vi "tx poulse host.vi"() -> ()   [LabVIEW 2021]
uses:
  <instrlib>/niUsrpRio/Config/v1/Host/Private/LO Source.ctl
  <vilib>/FPGAPlugInAG/USRP 294xR; 295xR 200 MSps/niLvFpga_Open_USRP 294xR; 295xR 200 MSps.vi
  <vilib>/rvi/interface/common/dynamic/niFpgaDynamicAddResources.vi
  <vilib>/Utility/error.llb/Error Cluster From Error Code.vi
  <vilib>/rvi/errors/niLvFpgaAdjustHostInterfaceError.vi
  <vilib>/rvi/interface/common/niFpgaWaitOnOcc.vi
  <vilib>/FPGAPlugInAG/Dynamic/niLvFpga_Close_Dynamic.vi
  <vilib>/rvi/interface/nirviOpenFPGA/nirviOpenFPGA.xnode
  FPGA Bitfiles/niUsrpRio200_XcvrTime.lvbitx
  <vilib>/rvi/interface/nirviMethod/nirviMethod.xnode
  <vilib>/rvi/interface/nirviReadWriteControl/nirviReadWriteControl.xnode
  <vilib>/rvi/interface/nirviCloseFPGA/nirviCloseFPGA.xnode
  <instrlib>/niUsrpRio/Config/v1/Host/niUsrpRio Config v1 Host.lvlib
  NiFpgaLv.dll
  <vilib>/rvi/interface/Simulation/niFpgaSimulationCallBeginRW.vi
  <vilib>/FPGAPlugInAG/Dynamic/niLvFpga_WriteFifo_Dynamic.vi
  <vilib>/rvi/errors/niLvFpgaMergeErrorWithErrorCode.vi
  <vilib>/FPGAPlugInAG/Dynamic/niLvFpga_ConfigureFifo_Dynamic.vi
panel:
  out "tx free":bool[](array[boolean])
  in  "analog file 3":path=path "C:/Users/NI/Documents/chaim/chaim_rx/chaim_data/good morning.wav"
  in  "analog file 2":path=path "C:/Users/NI/Documents/chaim/chaim_rx/chaim_data/good morning.wav"
  in  "analog file 1":path=path "C:/Users/NI/Documents/chaim/chaim_rx/chaim_data/good morning.wav"
  out "# pulse sent to FPGA":dbl
  out "pulse Tx by FPGA":u32
  out "fpga clock":dbl
  in  "tdms pulse istraction file path":path=path "C:/Users/NI/Documents/chaim/chaim_rx/chaim_data/pulses.tdms"
  in  "stop":bool
  in  "gain 0":dbl=-20.0 format="%#_6p"
  in  "Tx. frequency 0":dbl=2000000000.0 format="%#_6p"
  # "pulse transmitter"
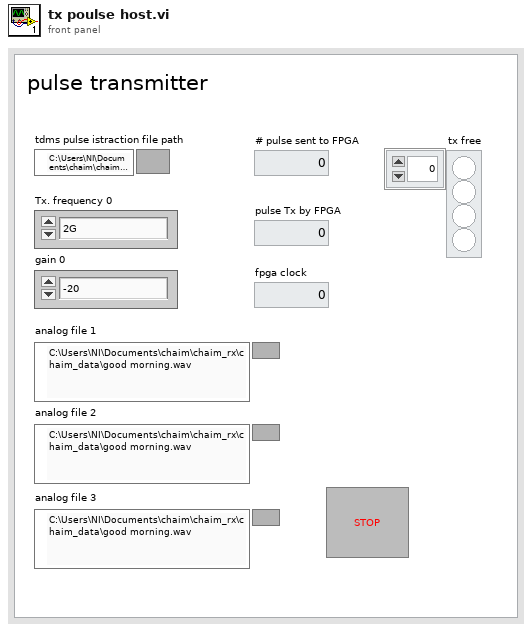
[diagram p1: front panel]
types:
  T1 = enum16{"open", "open or create", "create or replace", "create", "open (read-only)"}
  T2 = typedef "niUsrpRio Config v1 Host.lvlib/LO Source.ctl" = enum16{"Internal", "Companion", "External", "Reimport"}
  T3 = typedef "niUsrpRio Config v1 Host.lvlib/niUsrpRio Session.ctl" = cluster{"FPGA Interface":refnum<k20>, "RIO Interface Number":u32, "Data Clock Rate":u32, "FPGA Data Clock Rate":u32, "Global Settings Register Bus":T4, "Radio 0 Settings Register Bus":T4, "Radio 1 Settings Register Bus":T4, "Radio Settings Bus Semaphore":T5, "DB Queues":T6[], "Characterization Data Valid?":bool, "EEPROM Header":T7, "Device Data Header":T8, "EEPROM Characterization Header":T9, "Characterization Data":T10[], "FPGA Current Version":u32, "FPGA Oldest Compatible Version":u32, "Fixed Logic Current Version":u32, "Fixed Logic Oldest Compatible Version":u32, "FPGA Radio Settings Bus Current Version":u32, "FPGA Radio Settings Bus Oldest Compatible Version":u32, "FPGA Board Config Current Version":u32, "FPGA Board Config Oldest Compatible Version":u32, "Daughterboard Clock Rate":u32, "daughterboard configuration session handles":u64[]}
  T4 = typedef "niInstr Register Bus v0 Host.lvlib/Register Bus Session.ctl" = refnum<queue>
  T5 = typedef "Semaphore RefNum" = refnum<k1>
  T6 = typedef "niUsrpRio Config v1 Host.lvlib/DB Queue Reference.ctl" = refnum<queue>
  T7 = typedef "niUsrpRio Config v1 Host.lvlib/EEPROM Header.ctl" = cluster{"Checksum":u32, "Product Code":u16, "Hardware Current Version":u16, "Hardware Oldest Compatible Version":u16, "EEPROM Map Current Version":u16, "EEPROM Map Oldest Compatible Version":u16, "User Password":string, "Pointer to Factory Header":u32, "Pointer to User Header":u32, "Recommended Interval":u16, "Number of Reserved Bytes":i32, "Number of Daughterboards":u8, "Daughterboard IDs":u16[], "Daughterboard Serial Numbers":string[]}
  T8 = typedef "niUsrpRio Config v1 Host.lvlib/EEPROM Device Data Header.ctl" = cluster{"Checksum":u32, "Number of Channels":u8, "Number of Gain Settings":u16[], "Pointer to Characterization Data":u32[], "Number of Reserved Bytes":i32, "Number of Frequencies":u16[]}
  T9 = typedef "niUsrpRio Config v1 Host.lvlib/EEPROM Characterization Header.ctl" = cluster{"Checksum":u32, "Date":timestamp, "Temperature":sgl, "Misc. Info":string, "Pointer to Device Data Header":u32, "Number of Reserved Bytes":i32}
  T10 = typedef "niUsrpRio Config v1 Host.lvlib/Characterization Data.ctl" = cluster{"Gains[dB]":dbl[], "Frequencies [Hz]":dbl[], "IQ Imbalance Table":T11[], "Measured Gains[dB]":dbl[][]}
  T11 = typedef "niUsrpRio Config v1 Host.lvlib/IQ Imbalance.ctl" = cluster{"Gain Imbalance [linear]":dbl, "Phase Imbalance [radians]":dbl, "Offset":cdb}
  T12 = cluster{"gain I":fxp<+/-,24,3>, "gain Q":fxp<+/-,24,3>}
  T13 = typedef "niInstr DSP v1 Shared.lvlib/IQ Impairments.ctl" = cluster{"inline gain I":fxp<+/-,18,1>, "inline gain Q":fxp<+/-,18,1>, "cross gain I":fxp<+/-,18,1>, "cross gain Q":fxp<+/-,18,1>, "pre-gain offset I":fxp<+/-,18,1>, "pre-gain offset Q":fxp<+/-,18,1>, "post-gain offset I":fxp<+/-,18,1>, "post-gain offset Q":fxp<+/-,18,1>}
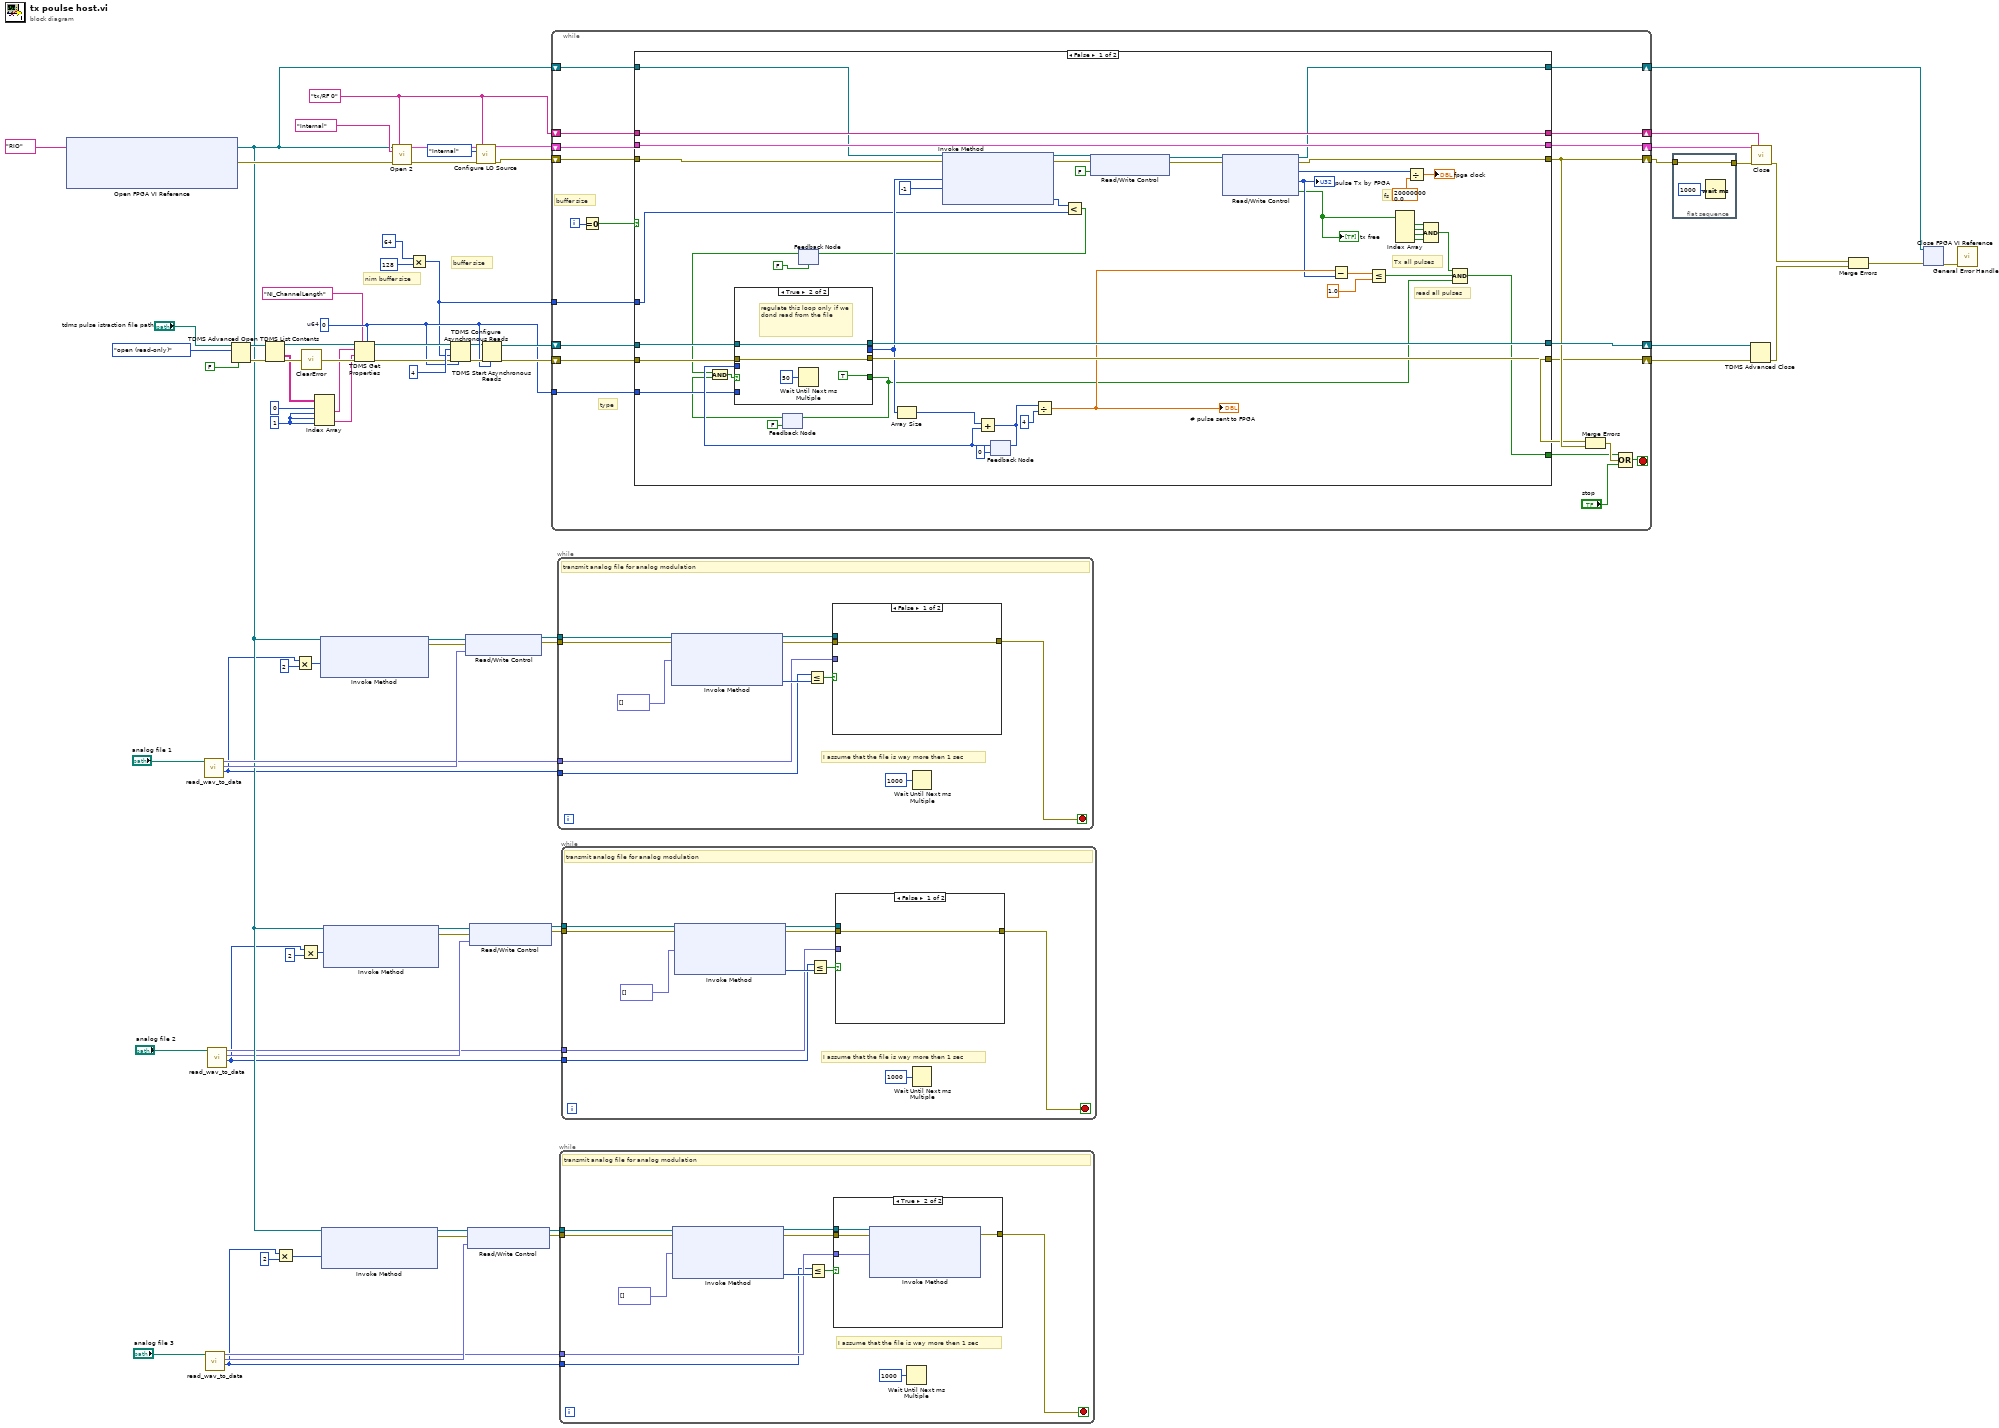
[diagram p0: block diagram]
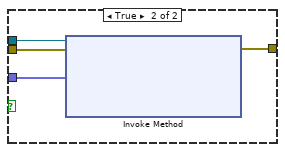
[diagram p3: hidden frame]
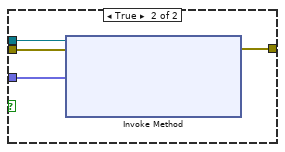
[diagram p4: hidden frame]
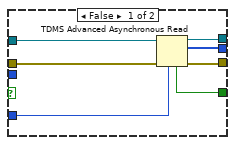
[diagram p5: hidden frame]
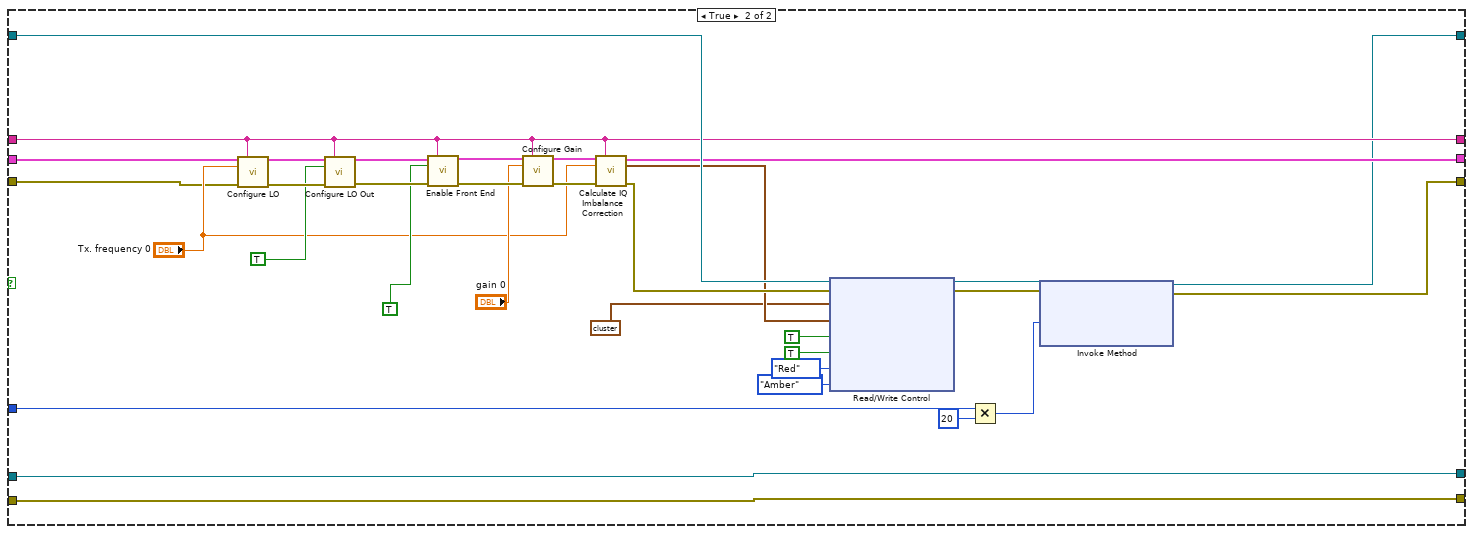
[diagram p6: hidden frame]
diagram:
  w46 = 1 ("disabled index (col)")
  w42 = u64 0  # u64
  w73 = "tx/RF 0" ("scope")
  # "buffer size"
  # "nim buffer size"
  n1 = xnode ("Open FPGA VI Reference")("resource name"=tag "RIO") -> ("FPGA VI Reference Out"=w15:refnum<k20>, "error out"=w39:errorcluster)  [unwired: 1 in]
  n2 = call "read_wav_to_data.vi"("path"="analog file 1") -> ("sampels on file"=w3:i32, "UP SAMPLE RATE"=w29:fxp<+,48,1>, "wav file out"=w28:fxp<+/-,18,1>[])  [unwired: 8 in]
  n3 = call "read_wav_to_data.vi"("path"="analog file 3") -> ("sampels on file"=w5:i32, "UP SAMPLE RATE"=w8:fxp<+,48,1>, "wav file out"=w7:fxp<+/-,18,1>[])  [unwired: 8 in]
  n4 = call "read_wav_to_data.vi"("path"="analog file 2") -> ("sampels on file"=w6:i32, "UP SAMPLE RATE"=w14:fxp<+,48,1>, "wav file out"=w11:fxp<+/-,18,1>[])  [unwired: 8 in]
  n5 = TDMS Advanced Open(6:FALSE ("Disable Buffering? (T)"), 10:T1."open (read-only)" ("Operation"), 11:"tdms pulse istraction file path") -> (0:w56:errorcluster, 3:w49:refnum<k34>)  [unwired: 2 in, 1 out]
  n6 = TDMS List Contents(4:w56, 7:w49) -> (0:w54:errorcluster, 1:w45:string[][], 3:w50:refnum<k34>)  [unwired: 1 in, 1 out]
  n7 = Multiply(x=w5, y=2) -> (x*y=w18:i32)
  n8 = Multiply(x=w3, y=2) -> (x*y=w32:i32)
  n9 = Multiply(x=w6, y=2) -> (x*y=w23:i32)
  n10 = call <vilib>:"ClearError.vi"("error in (no error)"=w54) -> ("error out"=w57:errorcluster)
  n11 = Index Array(array=w45, index (row) #1=0 ("index (row)"), index (col) #1=w46, index (row) #2=w46, index (col) #2=w46) -> (element #1=w44:string, element #2=w43:string)
  n12 = xnode ("Invoke Method")("FPGA VI Reference In"=w15, "Requested Depth"=w32) -> ("FPGA VI Reference Out"=w31:refnum<k20>, "error out"=w30:errorcluster)  [unwired: 1 in, 1 out]
  n13 = xnode ("Invoke Method")("FPGA VI Reference In"=w15, "Requested Depth"=w18) -> ("FPGA VI Reference Out"=w10:refnum<k20>, "error out"=w9:errorcluster)  [unwired: 1 in, 1 out]
  n14 = xnode ("Invoke Method")("FPGA VI Reference In"=w15, "Requested Depth"=w23) -> ("FPGA VI Reference Out"=w13:refnum<k20>, "error out"=w12:errorcluster)  [unwired: 1 in, 1 out]
  n15 = TDMS Get Properties(5:w42, 7:"NI_ChannelLength" ("property name"), 8:w57, 9:w43, 10:w44, 11:w50) -> (0:w55:errorcluster, 3:w48:refnum<k34>)  [unwired: 4 out]
  n16 = call <instrlib>:"Open 2.vi"("fpga ref"=w15, "scope"=w73, "Reference Frequency Source"="Internal", "error in"=w39) -> ("niUsrpRio Session (out)"=w65:T3, "error out"=w75:errorcluster)  [unwired: 10 in]
  n17 = Multiply(x=u32 64, y=u32 128 ("buffer size")) -> (x*y=w35:u32)
  n18 = TDMS Configure Asynchronous Reads(6:w42, 8:w55, 9:w35, 10:u32 4 ("Number of Buffers (4)"), 11:w48) -> (0:w59:errorcluster, 3:w41:refnum<k34>)  [unwired: 1 in]
  n19 = xnode ("Read/Write Control")("FPGA VI Reference In"=w31, "error in"=w30, "UP SAMPLE RATE"=w29) -> ("FPGA VI Reference Out"=w27:refnum<k20>, "error out"=w26:errorcluster)
  n20 = xnode ("Read/Write Control")("FPGA VI Reference In"=w10, "error in"=w9, "UP SAMPLE RATE 3"=w8) -> ("FPGA VI Reference Out"=w17:refnum<k20>, "error out"=w16:errorcluster)
  n21 = xnode ("Read/Write Control")("FPGA VI Reference In"=w13, "error in"=w12, "UP SAMPLE RATE 2"=w14) -> ("FPGA VI Reference Out"=w24:refnum<k20>, "error out"=w25:errorcluster)
  n22 = call <instrlib>:"Configure LO Source.vi"("niUsrpRio Session"=w65, "scope"=w73, "lo source"=LO_Source."Internal", "error in"=w75) -> ("niUsrpRio Session (out)"=w72:T3, "error out"=w71:errorcluster)  [unwired: 10 in]
  n23 = TDMS Start Asynchronous Reads(6:w42, 8:w59, 11:w41) -> (0:w51:errorcluster, 3:w52:refnum<k34>)  [unwired: 1 in]
  n24 = while {
    shift-right: [w82] -> w2
    shift-left: w71 -> [w95]
    shift-right: [w93] -> w70
    shift-left: w72 -> [w96]
    shift-right: [w92] -> w66
    shift-left: w15 -> [w94]
    shift-right: [w90] -> w69
    shift-left: w73 -> [w91]
    shift-right: [w85] -> w64
    shift-left: w52 -> [w87]
    shift-right: [w81] -> w63
    shift-left: w51 -> [w86]
    tunnel: w42 -> [w84]
    tunnel: w35 -> [w83]
    i -> [w88]
    stop <- w78 stop-if-true
    # "buffer size"
    # "type"
    n25 = Equal To 0?(x=w88) -> (x = 0?=w89:bool)
    n26 = case shown="False" w89 {
      tunnel: w96 -> [w142 w175]
      tunnel: w95 -> [w136 w174]
      tunnel: w94 -> [w135 w173]
      tunnel: [w142 w171] -> w93
      tunnel: [w111 w161] -> w92
      tunnel: [w110 w160] -> w82
      tunnel: w91 -> [w143 w170]
      tunnel: [w143 w170] -> w90
      tunnel: w87 -> [w134 w165]
      tunnel: w86 -> [w133 w164]
      tunnel: [w132 w165] -> w85
      tunnel: [w131 w164] -> w81
      tunnel: w84 -> [w125 _]
      tunnel: w83 -> [w122 w159]
      tunnel: [w104 _] -> w77
      frame False {
        # "fs"
        # "read all pulses"
        # "Tx all pulses"
        n27 = feedback #1(FALSE ("end of file?")) -> (w121:bool)
        n28 = feedback #2(FALSE) -> (w120:bool)
        n29 = Compound Arithmetic op=AND(w120, w121) -> (w117:bool)
        n30 = feedback #3(u32 0) -> (w129:u32)
        n31 = case shown="True" w117 {
          tunnel: w134 -> [w150 w154]
          tunnel: w133 -> [w145 w153]
          tunnel: [w149 w154] -> w132
          tunnel: [w146 w153] -> w131
          tunnel: [w147 _] -> w130
          tunnel: [w148 TRUE ("end of file?")] -> w103
          tunnel: w129 -> [_ _]
          tunnel: w125 -> [w144 _]
          frame False {
            n32 = TDMS Advanced Asynchronous Read(6:w144, 8:w145, 11:w150) -> (0:w146:errorcluster, 2:w147:u64[], 3:w149:refnum<k34>, 4:w148:bool)
          }
          frame True {
            # "regulate this loop only if we dond read from the file"
            n33 = Wait Until Next ms Multiple(millisecond multiple=u32 50) -> ()  [unwired: 1 out]
          }
        }
        n34 = feedback-in #1(w103) -> ()
        n35 = Array Size(array=w130) -> (size(s)=w127:i32)
        n36 = xnode ("Invoke Method")("FPGA VI Reference In"=w135, "error in"=w136, "Data"=w130, "Timeout (ms)"=-1) -> ("FPGA VI Reference Out"=w139:refnum<k20>, "error out"=w140:errorcluster, "Empty Elements Remaining"=w123:u32)
        n37 = Add(x=w127, y=w129) -> (x+y=w116:u32)
        n38 = feedback-in #3(w116) -> ()
        n39 = Divide(x=w116, y=u32 4) -> (x/y=w109:dbl)
        "# pulse sent to FPGA" <- w109
        n40 = Less?(x=w123, y=w122) -> (x < y?=w119:bool)
        n41 = feedback-in #2(w119) -> ()
        n42 = xnode ("Read/Write Control")("FPGA VI Reference In"=w139, "error in"=w140, "reset system clock"=FALSE) -> ("FPGA VI Reference Out"=w138:refnum<k20>, "error out"=w137:errorcluster)
        n43 = xnode ("Read/Write Control")("FPGA VI Reference In"=w138, "error in"=w137) -> ("FPGA VI Reference Out"=w111:refnum<k20>, "error out"=w110:errorcluster, "fpga clock"=w113:u64, "pulse transmitted"=w108:u32, "tx free"=w102:bool[])
        "pulse Tx by FPGA" <- w108
        "tx free" <- w102
        n44 = Subtract(x=w109, y=w108) -> (x-y=w107:dbl)
        n45 = Less Or Equal?(x=w107, y=1.0) -> (x <= y?=w105:bool)
        n46 = Index Array(array=w102) -> (element #1=w101:bool, element #2=w100:bool, element #3=w99:bool, element #4=w98:bool)  [unwired: 4 in]
        n47 = Divide(x=w113, y=200000000.0) -> (x/y=→"fpga clock":dbl)
        n48 = Compound Arithmetic op=AND(w101, w100, w99, w98) -> (w97:bool)
        n49 = Compound Arithmetic op=AND(w97, w105, w103) -> (w104:bool)
      }
      frame True {
        n50 = call <instrlib>:"Configure LO.vi"("niUsrpRio Session"=w175, "scope"=w170, "frequency"="Tx. frequency 0", "error in"=w174) -> ("niUsrpRio Session (out)"=w187:T3, "error out"=w186:errorcluster)  [unwired: 8 in, 2 out]
        n51 = call <instrlib>:"Configure LO Out.vi"("niUsrpRio Session"=w187, "scope"=w170, "enable"=TRUE ("enable 0"), "error in"=w186) -> ("niUsrpRio Session (out)"=w184:T3, "error out"=w181:errorcluster)  [unwired: 10 in]
        n52 = call <instrlib>:"Enable Front End.vi"("niUsrpRio Session"=w184, "scope"=w170, "enable"=TRUE ("enable 0 2"), "error in"=w181) -> ("niUsrpRio Session (out)"=w183:T3, "error out"=w182:errorcluster)  [unwired: 10 in]
        n53 = call <instrlib>:"Configure Gain.vi"("niUsrpRio Session"=w183, "scope"=w170, "gain"="gain 0", "error in"=w182) -> ("niUsrpRio Session (out)"=w178:T3, "error out"=w177:errorcluster)  [unwired: 9 in, 1 out]
        n54 = call <instrlib>:"Calculate IQ Imbalance Correction.vi"("niUsrpRio Session"=w178, "scope"=w170, "frequency"="Tx. frequency 0", "error in"=w177) -> ("niUsrpRio Session (out)"=w171:T3, "IQ imbalance correction"=w167:T13, "error out"=w172:errorcluster)  [unwired: 8 in, 1 out]
        n55 = xnode ("Read/Write Control")("FPGA VI Reference In"=w173, "error in"=w172, "tx.gain.0"=T12 {"gain I"=1.0, "gain Q"=1.0}, "tx.impairments.0"=w167, "reset system clock"=TRUE, "RF 0/Tx/Enable"=TRUE, "LED/RF 0/TX1 RX1"=enum8{"Off", "Green", "Red", "Amber"}."Red", "LED/RF 1/TX1 RX1"=enum8{"Off", "Green", "Red", "Amber"}."Amber") -> ("FPGA VI Reference Out"=w163:refnum<k20>, "error out"=w162:errorcluster)
        n56 = Multiply(x=w159, y=u32 20) -> (x*y=w157:u32)
        n57 = xnode ("Invoke Method")("FPGA VI Reference In"=w163, "error in"=w162, "Requested Depth"=w157) -> ("FPGA VI Reference Out"=w161:refnum<k20>, "error out"=w160:errorcluster)  [unwired: 1 out]
      }
    }
    n58 = Merge Errors(w81, w82) -> (w79:errorcluster)
    n59 = Compound Arithmetic op=OR(w77, w79, "stop") -> (w78:bool)
  }
  n60 = while {
    tunnel: w3 -> [w193]
    tunnel: w28 -> [w192]
    tunnel: w27 -> [w191]
    tunnel: w26 -> [w190]
    stop <- w189 stop-if-true
    # "I assume that the file is way more then 1 sec"
    # "transmit analog file for analog modulation"
    n61 = xnode ("Invoke Method")("FPGA VI Reference In"=w191, "error in"=w190, "Data"=fxp<+/-,18,1>[] []) -> ("FPGA VI Reference Out"=w198:refnum<k20>, "error out"=w197:errorcluster, "Empty Elements Remaining"=w195:u32)  [unwired: 1 in]
    n62 = Less Or Equal?(x=w193, y=w195) -> (x <= y?=w194:bool)
    n63 = case shown="False" w194 {
      tunnel: [w199 w203] -> w189
      tunnel: w198 -> [_ w202]
      tunnel: w197 -> [w199 w201]
      tunnel: w192 -> [_ w200]
      frame False {
      }
      frame True {
        n64 = xnode ("Invoke Method")("FPGA VI Reference In"=w202, "error in"=w201, "Data"=w200) -> ("error out"=w203:errorcluster)  [unwired: 1 in, 2 out]
      }
    }
    n65 = Wait Until Next ms Multiple(millisecond multiple=u32 1000) -> ()  [unwired: 1 out]
  }
  n66 = while {
    tunnel: w17 -> [w209]
    tunnel: w16 -> [w208]
    tunnel: w7 -> [w206]
    tunnel: w5 -> [w205]
    stop <- w207 stop-if-true
    # "I assume that the file is way more then 1 sec"
    # "transmit analog file for analog modulation"
    n67 = xnode ("Invoke Method")("FPGA VI Reference In"=w209, "error in"=w208, "Data"=fxp<+/-,18,1>[] []) -> ("FPGA VI Reference Out"=w214:refnum<k20>, "error out"=w213:errorcluster, "Empty Elements Remaining"=w211:u32)  [unwired: 1 in]
    n68 = Less Or Equal?(x=w205, y=w211) -> (x <= y?=w210:bool)
    n69 = case shown="True" w210 {
      tunnel: [w215 w219] -> w207
      tunnel: w214 -> [_ w218]
      tunnel: w213 -> [w215 w217]
      tunnel: w206 -> [_ w216]
      frame False {
      }
      frame True {
        n70 = xnode ("Invoke Method")("FPGA VI Reference In"=w218, "error in"=w217, "Data"=w216) -> ("error out"=w219:errorcluster)  [unwired: 1 in, 2 out]
      }
    }
    n71 = Wait Until Next ms Multiple(millisecond multiple=u32 1000) -> ()  [unwired: 1 out]
  }
  n72 = while {
    tunnel: w24 -> [w225]
    tunnel: w25 -> [w224]
    tunnel: w11 -> [w222]
    tunnel: w6 -> [w221]
    stop <- w223 stop-if-true
    # "I assume that the file is way more then 1 sec"
    # "transmit analog file for analog modulation"
    n73 = xnode ("Invoke Method")("FPGA VI Reference In"=w225, "error in"=w224, "Data"=fxp<+/-,18,1>[] []) -> ("FPGA VI Reference Out"=w230:refnum<k20>, "error out"=w229:errorcluster, "Empty Elements Remaining"=w227:u32)  [unwired: 1 in]
    n74 = Less Or Equal?(x=w221, y=w227) -> (x <= y?=w226:bool)
    n75 = case shown="False" w226 {
      tunnel: [w231 w235] -> w223
      tunnel: w230 -> [_ w234]
      tunnel: w229 -> [w231 w233]
      tunnel: w222 -> [_ w232]
      frame False {
      }
      frame True {
        n76 = xnode ("Invoke Method")("FPGA VI Reference In"=w234, "error in"=w233, "Data"=w232) -> ("error out"=w235:errorcluster)  [unwired: 1 in, 2 out]
      }
    }
    n77 = Wait Until Next ms Multiple(millisecond multiple=u32 1000) -> ()  [unwired: 1 out]
  }
  n78 = flat-sequence {
    tunnel: w2 -> [w237]
    tunnel: [w237] -> w1
    frame #0 {
      n79 = Wait (ms)(milliseconds to wait=u32 1000) -> ()  [unwired: 1 out]
    }
  }
  n80 = TDMS Advanced Close(8:w63, 11:w64) -> (0:w62:errorcluster)  [unwired: 2 in, 1 out]
  n81 = call <instrlib>:"Close.vi"("niUsrpRio Session"=w70, "scope"=w69, "error in"=w1) -> ("error out"=w68:errorcluster)  [unwired: 11 in, 1 out]
  n82 = Merge Errors(w68, w62) -> (w67:errorcluster)
  n83 = xnode ("Close FPGA VI Reference")("FPGA VI Reference In"=w66, "error in"=w67) -> ("error out"=w4:errorcluster)
  n84 = call <vilib>:"General Error Handler.vi"("error in (no error)"=w4) -> ()  [unwired: 10 in, 5 out]
